vi "Send Integral.vi"(0 "Message Enqueuer":refnum<class "Message Enqueuer.lvclass">, 1 "-t1":dbl[unit], 2 "t100":dbl[unit], 5 "error in (no error)":errorcluster, 6 "Message Priority (Normal)":T1=enum."Normal") -> (14 "Message Enqueuer out":refnum<class "Message Enqueuer.lvclass">, 19 "error out":errorcluster)   [LabVIEW 2015, in "KIT-QA.lvlib" / "Integral Msg.lvclass"]
doc: "Sends the <B>KIT-QA.lvlib:Integral Msg.lvclass</B> message.\n\n<B>KIT-QA.lvlib:KIT-QA.lvclass:Integral.vi</B> Description:\n\nPiotr's Integral"
uses:
  Integral Msg.lvclass
  <vilib>/ActorFramework/Message Enqueuer/Message Enqueuer.lvclass
  <vilib>/ActorFramework/Message Enqueuer/Message Priority.ctl
  Integral Msg.lvclass/Integral Msg.ctl
  <vilib>/ActorFramework/Message Enqueuer/Message Enqueuer.lvclass/Message Enqueuer.ctl
  <vilib>/ActorFramework/Message Priority Queue/Priority Enqueue.vi
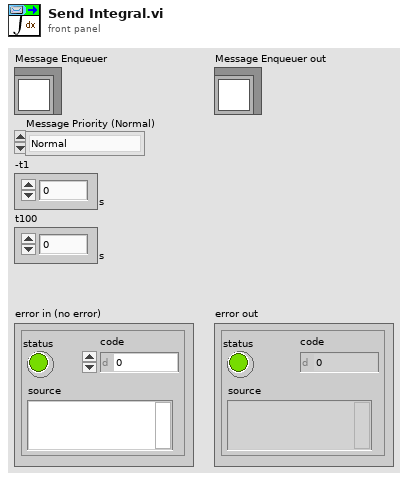
[diagram p1: front panel]
types:
  T1 = typedef "Actor Framework.lvlib/Message Enqueuer.lvclass/Message Priority.ctl" = enum16{"Low", "Normal", "High"}
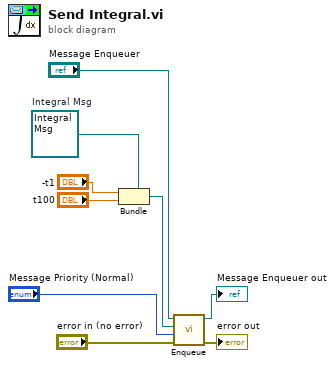
[diagram p0: block diagram]
diagram:
  w3 = refnum<class "Integral Msg.lvclass"> refnum  # Integral Msg
  n1 = Bundle(cluster=w3, "-t1", "t100") -> (w6:refnum<class "Integral Msg.lvclass">)
  n2 = call <vilib>:"Enqueue.vi"("error in (no error)"="error in (no error)", "Message Priority (Normal)"="Message Priority (Normal)", "Message"=w6, "Message Enqueuer in"="Message Enqueuer") -> ("error out"=→"error out":errorcluster, "Message Enqueuer out"=→"Message Enqueuer out":refnum<class "Message Enqueuer.lvclass">)  [unwired: 6 in]
